vi "default ARM MACRO pgm.vi"(8 "error in (no error)":errorcluster) -> (0 "error out":errorcluster)   [LabVIEW 2020]
doc: "This is meant to be a default starting VI for an arm macro. Please SAVEAS something else.\n\nTHIS is the description. Go to the FRONT PAGE and rt-click the icon. \nSelect VI properties.\nin Category, select Documentation."
uses:
  ctrl ARM MACRO ENTRY.ctl
  Robot Global Data.vi
panel:
  out "HANGAR BARS":T1={"LOW BAR AG"=48.75, "MID BAR AG"=60.25, "HIGH BAR AG"=75.625, "TRAV BAR AG"=91.0, "BAR OD"=1.66, "SPACING"=24.0}
  out "ARM Climber range":T2={"MIN"=0.0, "MAX"=22.5, "convert climber inches to tics"=18192.520379, "INITIALIZE"=-0.0625} {"convert climber inches to tics" format="%.6g"}
  out "ARM angle range":T3={"MIN"=-3.5, "MAX"=4.5, "convert arm inches to revs"=42.857, "convert arm inches to degrees"=4.96493} {"convert arm inches to degrees" format="%.6g"; "convert arm inches to revs" format="%.6g"}
  out "ARM DIMS":T4={"HOOK CTR LENGTH LEFT"=39.075, "HOOK CTR LENGTH RIGHT"=42.7, "HOOK DEPTH"=2.0, "HOOK ID"=1.875, "SHOULDER PIN AG"=6.875, "ARM DIFF RT-LEFT"=3.625}
  in  "Array":T6(array[cluster]) {"RIGHT"."Angle"."speed" min=0.0 max=1.0 format="%_3g"; "RIGHT"."Angle"."ARM ANGLE (deg)" format="%.3g"; "RIGHT"."Climber"."CLIMBER STROKE (in)" format="%_5g"; "RIGHT"."Climber"."speed" min=0.0 max=1.0 format="%_3g"; "LEFT"."Angle"."speed" min=0.0 max=1.0 format="%_3g"; "LEFT"."Angle"."ARM ANGLE (deg)" format="%.3g"; "LEFT"."Climber"."CLIMBER STROKE (in)" format="%_5g"; "LEFT"."Climber"."speed" min=0.0 max=1.0 format="%_3g"}
  # "descr"
  # "22-03-14 measured arm lengths:\nat 0% stroke, the inside hook openings were\nLEFT = 40.375\"  and RIGHT = 44.0\"\nwrt top of the shoulder arm plate"
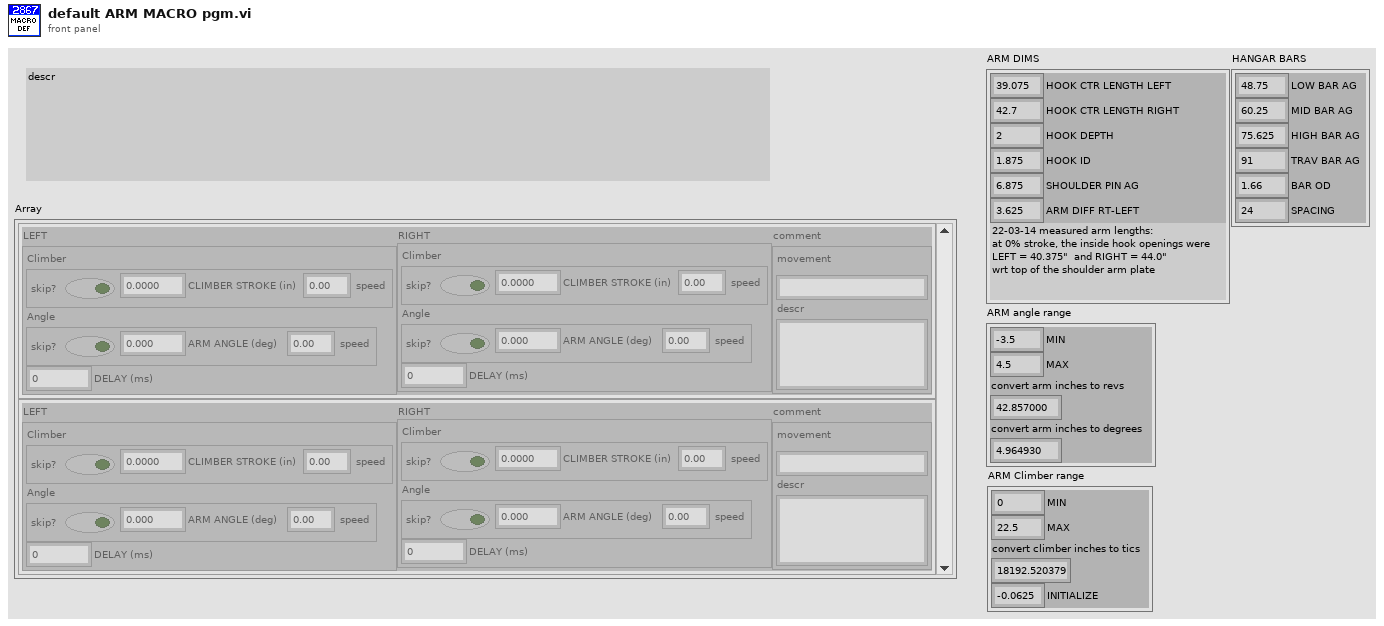
[diagram p1: front panel]
types:
  T1 = cluster{"LOW BAR AG":dbl, "MID BAR AG":dbl, "HIGH BAR AG":dbl, "TRAV BAR AG":dbl, "BAR OD":dbl, "SPACING":dbl}
  T2 = cluster{"MIN":dbl, "MAX":dbl, "convert climber inches to tics":dbl, "INITIALIZE":dbl}
  T3 = cluster{"MIN":dbl, "MAX":dbl, "convert arm inches to revs":dbl, "convert arm inches to degrees":dbl}
  T4 = cluster{"HOOK CTR LENGTH LEFT":dbl, "HOOK CTR LENGTH RIGHT":dbl, "HOOK DEPTH":dbl, "HOOK ID":dbl, "SHOULDER PIN AG":dbl, "ARM DIFF RT-LEFT":dbl}
  T5 = typedef "ctrl ARM MACRO ENTRY.ctl" = cluster{"Climber":cluster{"skip?":bool, "CLIMBER STROKE (in)":dbl, " speed":dbl}, "Angle":cluster{"skip?":bool, "ARM ANGLE (deg)":dbl, " speed":dbl}, "DELAY (ms)":u32}
  T6 = cluster{"LEFT":T5, "RIGHT":T5, "comment":cluster{"movement":string, "descr":string}}[]
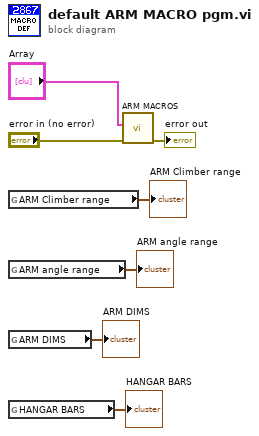
[diagram p0: block diagram]
diagram:
  n1 = global read "Robot Global Data.vi" "ARM Climber range"() -> (→"ARM Climber range":T2)
  n2 = global read "Robot Global Data.vi" "ARM angle range"() -> (→"ARM angle range":T3)
  n3 = global read "Robot Global Data.vi" "ARM DIMS"() -> (→"ARM DIMS":T4)
  n4 = global read "Robot Global Data.vi" "HANGAR BARS"() -> (→"HANGAR BARS":T1)
  n5 = call "ARM MACROS.vi"("error in (no error)"="error in (no error)", "Array"="Array") -> ("error out"=→"error out":errorcluster)  [unwired: 9 in]
